vi "SRV_Sensor PARSE_#NB.vi"(0 "Return Data":string, 11 "error in (no error)":errorcluster) -> (3 "Sensor View Indicator Names":T1, 6 "Values (U8)":u8[](array[numeric]) format="%.0x", 15 "error out":errorcluster)   [LabVIEW 2009]
uses:
  SRV_Sensors Names.ctl
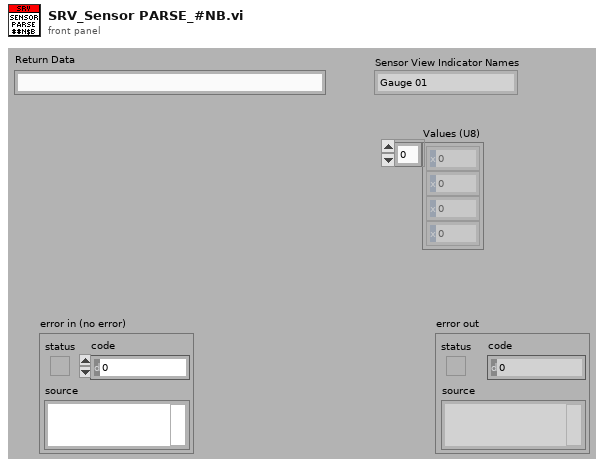
[diagram p1: front panel]
types:
  T1 = typedef "SRV_Sensors Names.ctl" = enum16{"Gauge 01", "Gauge 02", "Gauge 03", "Gauge 04", "Meter 01", "Meter 02", "Meter 03", "Meter 04", "Numeric 01", "Numeric 02", "Numeric 03", "Numeric 04", "Numeric 05", "Numeric 06", "Numeric 07", "Numeric 08", "Boolean 01", "Boolean 02", "Boolean 03", "Boolean 04", "Boolean 05", "Boolean 06", "Boolean 07", "Boolean 08", "Boolean 09", "Boolean 10", "Boolean 11", "Boolean 12", "Boolean 13", "Boolean 14", "Boolean 15", "Boolean 16", "Boolean 17", "Boolean 18", "Boolean 19", "Boolean 20", "Boolean 21", "Boolean 22", "Boolean 23", "Boolean 24", "Boolean 25", "Boolean 26", "Boolean 27", "Boolean 28", "Boolean 29", "Boolean 30", "Boolean 31", "Boolean 32"}
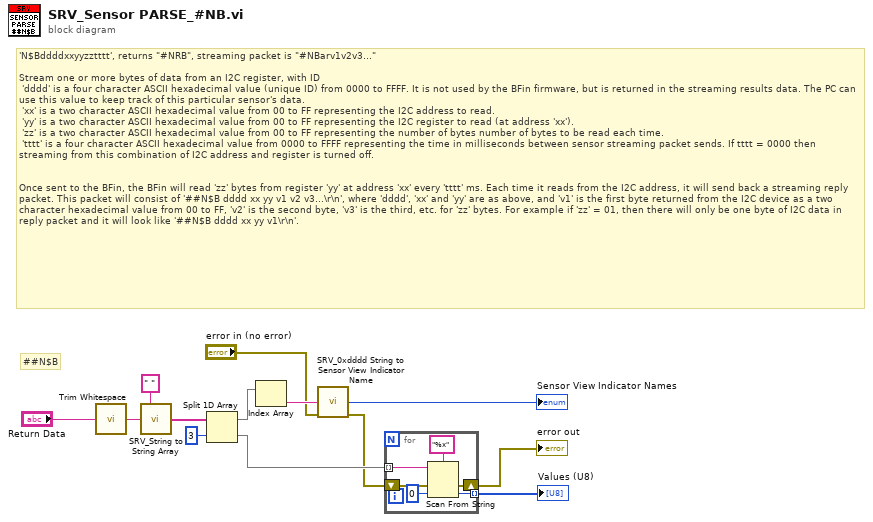
[diagram p0: block diagram]
diagram:
  # "##N$B"
  # "'N$Bddddxxyyzztttt', returns \"#NRB\", streaming packet is \"#NBarv1v2v3…\"\n\nStream one or more bytes of data from an I2C register, with ID\n 'dddd' is a four character ASCII hexadecimal value (unique ID) from 0000 to FFFF. It is not used by the BFin firmware, but is returned in the streaming results data. The PC can use this value to keep track of this particular sensor's data.\n 'xx' is a two character ASCII hexadecimal value from 00 to FF representing the I2C address to read.\n 'yy' is a two character ASCII hexadecimal value from 00 to FF representing the I2C register to read (at address 'xx').\n 'zz' is a two character ASCII hexadecimal value from 00 to FF representing the number of bytes number of bytes to be read each time.\n 'tttt' is a four character ASCII hexadecimal value from 0000 to FFFF representing the time in milliseconds between sensor streaming packet sends. If tttt = 0000 then streaming from this combination of I2C address and register is turned off.\n\n\nOnce sent to the BFin, the BFin will read 'zz' bytes from register 'yy' at address 'xx' every 'tttt' ms. Each time it reads from the I2C address, it will send back a streaming reply packet. This packet will consist of '##N$B dddd xx yy v1 v2 v3...\\r\\n', where 'dddd', 'xx' and 'yy' are as above, and 'v1' is the first byte returned from the I2C device as a two character hexadecimal value from 00 to FF, 'v2' is the second byte, 'v3' is the third, etc. for 'zz' bytes. For example if 'zz' = 01, then there will only be one byte of I2C data in reply packet and it will look like '##N$B dddd xx yy v1\\r\\n'."
  n1 = call <vilib>:"Trim Whitespace.vi"("string"="Return Data") -> ("trimmed string"=w12:string)  [unwired: 1 in]
  n2 = call "SRV_String to String Array.vi"("Element Separator (,)"=" ", "String"=w12) -> ("String Array"=w10:string[])  [unwired: 13 in]
  n3 = Split 1D Array(array=w10, index=3) -> (first subarray=w8:string[], second subarray=w5:string[])
  n4 = Index Array(array=w8) -> (element=w7:string)  [unwired: 1 in]
  n5 = call "SRV_0xdddd String to Sensor View Indicator Name.vi"("dddd"=w7, "error in (no error)"="error in (no error)") -> ("Sensor View Indicator Names"=→"Sensor View Indicator Names":T1, "error out"=w2:errorcluster)  [unwired: 12 in]
  n6 = for {
    tunnel: w5 -> [w17] mode=indexing
    tunnel: [w16] -> w4 mode=indexing
    shift-right: [w14] -> w1
    shift-left: w2 -> [w15]
    n7 = Scan From String(format string="%x", input string=w17, error in=w15, default 1=u8 0) -> (error out=w14:errorcluster, output 1=w16:u8)  [unwired: 1 in, 2 out]
  }
  "Values (U8)" <- w4
  "error out" <- w1
